vi "test.vi"() -> ()   [LabVIEW 2017]
panel:
  out "Data Name 3":string
  out "Data Name 2":string
  out "Data Name":string
  in  "Numeric":dbl
  in  "error in (no error)":errorcluster
  in  "Cluster":cluster{"Numeric":dbl}
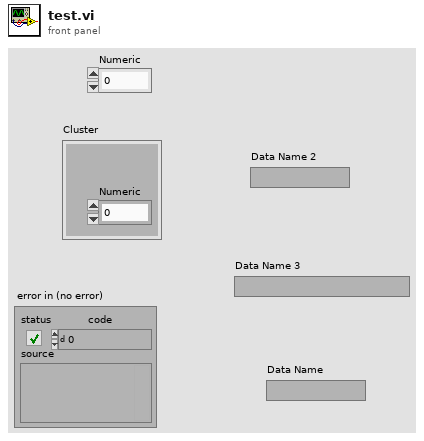
[diagram p1: front panel]
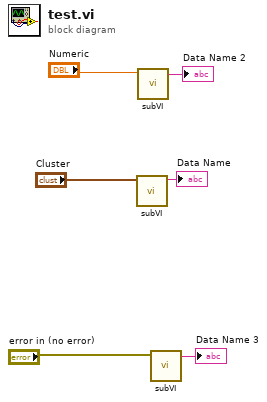
[diagram p0: block diagram]
diagram:
  n1 = call "subVI.vi"("Variant"="Cluster") -> ("Data Name"=→"Data Name":string)  [unwired: 10 in]
  n2 = call "subVI.vi"("Variant"="Numeric") -> ("Data Name"=→"Data Name 2":string)  [unwired: 10 in]
  n3 = call "subVI.vi"("Variant"="error in (no error)") -> ("Data Name"=→"Data Name 3":string)  [unwired: 10 in]
